vi "piano.vi"() -> ()   [LabVIEW 2016]
uses:
  <vilib>/userdefined/High Color/IMAQdx.ctl
  <vilib>/vision/driver/NI_Vision_Acquisition_Software.lvlib
  <vilib>/measure/NI_MABase.lvlib
panel:
  in  "Number of Erosion (Adv. Morphology 2)":i32=4
  in  "Threshold dedos":cluster{"Lower value":sgl, "Upper value":sgl}={"Lower value"=0.0, "Upper value"=20.0}
  in  "Threshold teclas":cluster{"Lower value":sgl, "Upper value":sgl}={"Lower value"=85.0, "Upper value"=255.0}
  in  "calibración":dbl
  out "Image":T1(plugin-control)
  out "Array":string[](array[string])
  in  "Stop (F)":bool
  out "Image Out":T1(plugin-control)
  # "100"
  # "Base y cámara fija:\n1- Configurar Mask\n2-configurar trheshold teclas blancas\n3-configurar threshold dedos\n4-configurar calibración (separación tolerable en pixeles\nde los centros de masa tecla y dedo)\n5-configurar número de teclas en código y orden de C a B"
  # "0"
  # "42"
  # "85"
  # "255"
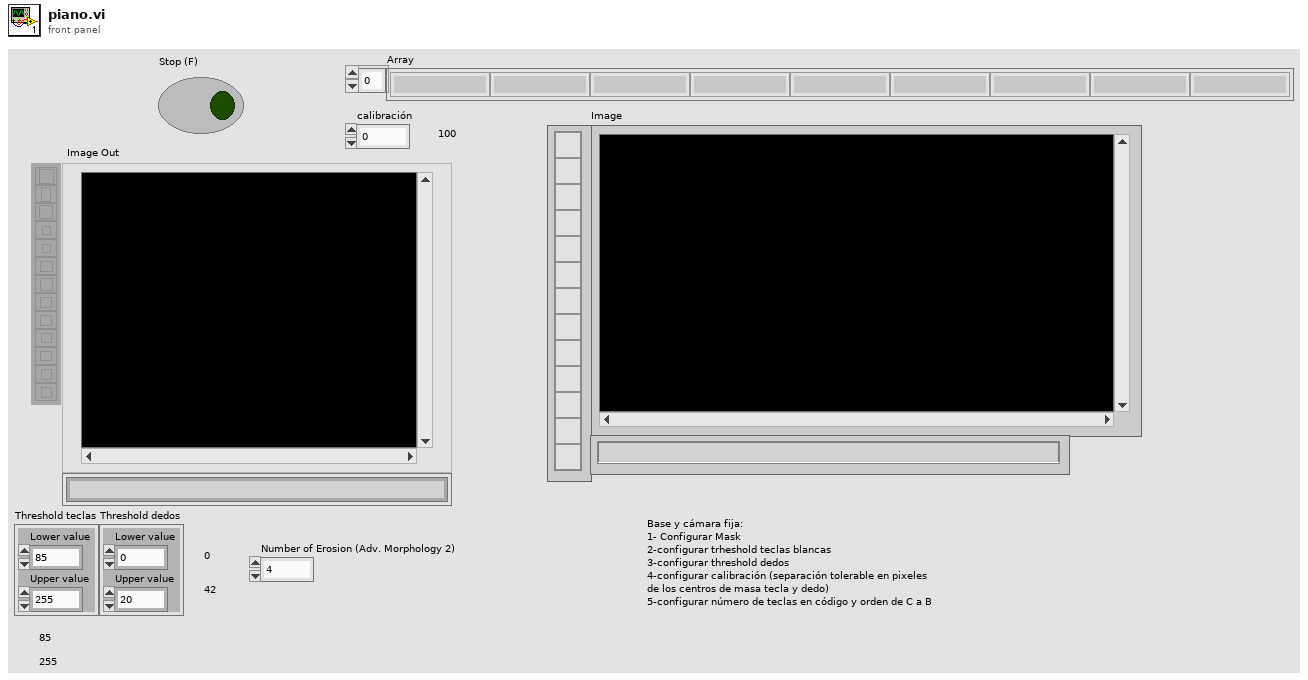
[diagram p1: front panel]
types:
  T1 = typedef "IMAQ Image.ctl" = refnum<image>
  T2 = typedef "Image Type" = u32
  T3 = typedef "IMAQdx.ctl" = refnum<k21>
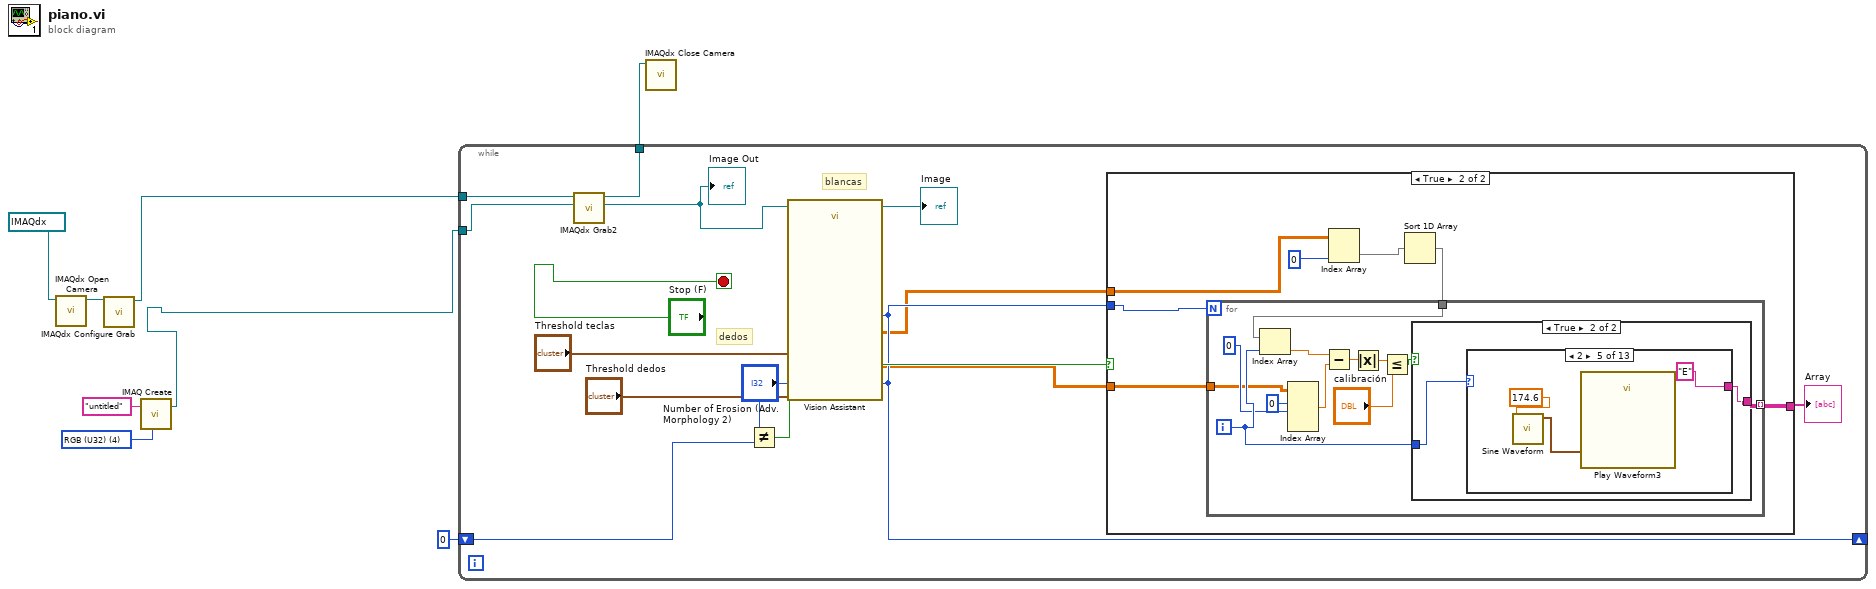
[diagram p0: block diagram]
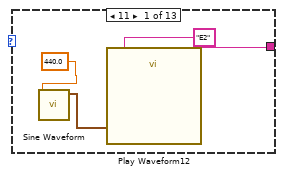
[diagram p4: hidden frame]
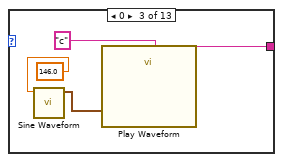
[diagram p6: hidden frame]
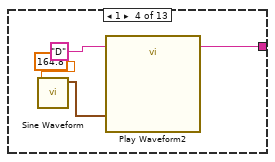
[diagram p7: hidden frame]
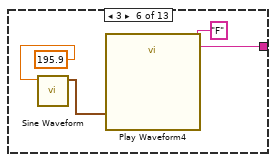
[diagram p8: hidden frame]
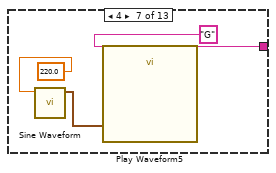
[diagram p9: hidden frame]
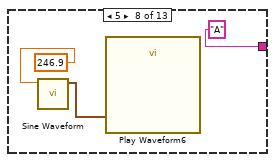
[diagram p10: hidden frame]
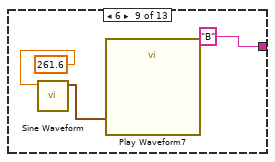
[diagram p11: hidden frame]
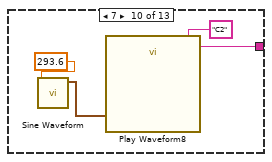
[diagram p12: hidden frame]
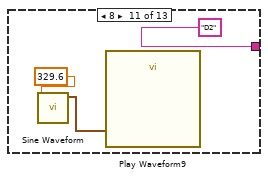
[diagram p13: hidden frame]
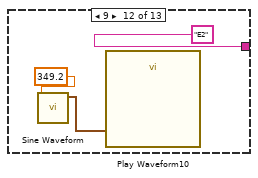
[diagram p14: hidden frame]
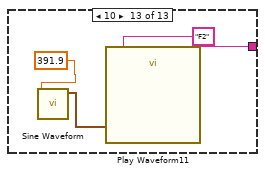
[diagram p15: hidden frame]
diagram:
  w1 = T2 4 items=["Grayscale (U8)", "Grayscale (I16)", "Grayscale (SGL)", "Complex (CSG)", "RGB (U32)", "HSL (U32)", "RGB (U64)", "Grayscale (U16)"] ("Image Type")
  n1 = call <vilib>:"IMAQdx Open Camera.vi"("Session In"=T3 "cam2") -> ("Session Out"=w8:T3)  [unwired: 9 in, 1 out]
  n2 = call <vilib>:"IMAQdx Configure Grab.vi"("Session In"=w8) -> ("Session Out"=w4:T3)  [unwired: 9 in, 1 out]
  n3 = call "IMAQ Create"("Image Name"="untitled", "Image Type"=w1) -> ("New Image"=w3:T1)  [unwired: 3 in, 1 out]
  n4 = while {
    tunnel: w4 -> [w19]
    tunnel: [w18] -> w7
    tunnel: w3 -> [w17]
    shift-right: [w15] -> _
    shift-left: 0 ("Number of Particles (Particle Analysis 1)") -> [w16]
    stop <- "Stop (F)" stop-if-true
    # "dedos"
    # "blancas"
    n5 = call <vilib>:"IMAQdx Grab2.vi"("Image In"=w17, "Session In"=w19) -> ("Image Out"=w13:T1, "Session Out"=w18:T3)  [unwired: 6 in, 2 out]
    "Image Out" <- w13
    n6 = call "Vision Assistant"("Image In"=w13, "Range (Threshold 1)"="Threshold teclas", "Range (Threshold 2)"="Threshold dedos", "Number of Erosion (Adv. Morphology 2)"="Number of Erosion (Adv. Morphology 2)") -> ("Image Out"=→"Image":T1, "Number of Particles (Particle Analysis 1)"=w15:i32, "Particle Measurements (Pixels) (Particle Analysis 1)"=w14:dbl[][], "Particle Measurements (Pixels) (Particle Analysis 2)"=w12:dbl[][])  [unwired: 18 in, 2 out]
    n7 = Not Equal?(x=w15, y=w16) -> (x != y?=w23:bool)
    n8 = case shown="True" w23 {
      tunnel: w14 -> [_ w27]
      tunnel: [_ w30] -> w22
      tunnel: w15 -> [_ w29]
      tunnel: w12 -> [_ w28]
      frame False {
      }
      frame True {
        n9 = Index Array(array=w27, index (col)=0 ("index (row)")) -> (element=w25:dbl[])  [unwired: 1 in]
        n10 = Sort 1D Array(array=w25) -> (sorted array=w24:dbl[])
        n11 = for {
          N: w29 -> [_]
          tunnel: [w42] -> w30 mode=indexing
          tunnel: w28 -> [w34]
          tunnel: w24 -> [w31]
          i -> [w41]
          n12 = Index Array(array=w31, index=w41) -> (element=w39:dbl)
          n13 = Index Array(array=w34, index (row) #1=0 ("disabled index (row)"), index (col) #1=0 ("index")) -> (element #1=w33:dbl)  [unwired: 2 in, 1 out]
          n14 = Subtract(x=w39, y=w33) -> (x-y=w38:dbl)
          n15 = Absolute Value(x=w38) -> (abs(x)=w36:dbl)
          n16 = Less Or Equal?(x=w36, y="calibración") -> (x <= y?=w37:bool)
          n17 = case shown="True" w37 {
            tunnel: w41 -> [_ w44]
            tunnel: [_ w43] -> w42
            frame False {
            }
            frame True {
              n18 = case shown="2" w44 {
                tunnel: ["E2" _ "c" "D" "E" "F" "G" "A" "B" "C2" "D2" "E2" "F2"] -> w43
                frame 11 {
                  n19 = call <vilib>:"Sine Waveform.vi"("frequency"=440.0) -> ("signal out"=w47:waveform(dbl))  [unwired: 9 in, 1 out]
                  n20 = call "Play Waveform12"("Data"=w47) -> ()  [unwired: 18 in, 1 out]
                }
                frame 12, Default {
                }
                frame 0 {
                  n21 = call <vilib>:"Sine Waveform.vi"("frequency"=146.0) -> ("signal out"=w48:waveform(dbl))  [unwired: 9 in, 1 out]
                  n22 = call "Play Waveform"("Data"=w48) -> ()  [unwired: 18 in, 1 out]
                }
                frame 1 {
                  n23 = call <vilib>:"Sine Waveform.vi"("frequency"=164.8) -> ("signal out"=w52:waveform(dbl))  [unwired: 9 in, 1 out]
                  n24 = call "Play Waveform2"("Data"=w52) -> ()  [unwired: 18 in, 1 out]
                }
                frame 2 {
                  n25 = call <vilib>:"Sine Waveform.vi"("frequency"=174.6) -> ("signal out"=w55:waveform(dbl))  [unwired: 9 in, 1 out]
                  n26 = call "Play Waveform3"("Data"=w55) -> ()  [unwired: 18 in, 1 out]
                }
                frame 3 {
                  n27 = call <vilib>:"Sine Waveform.vi"("frequency"=195.9) -> ("signal out"=w58:waveform(dbl))  [unwired: 9 in, 1 out]
                  n28 = call "Play Waveform4"("Data"=w58) -> ()  [unwired: 18 in, 1 out]
                }
                frame 4 {
                  n29 = call <vilib>:"Sine Waveform.vi"("frequency"=220.0) -> ("signal out"=w61:waveform(dbl))  [unwired: 9 in, 1 out]
                  n30 = call "Play Waveform5"("Data"=w61) -> ()  [unwired: 18 in, 1 out]
                }
                frame 5 {
                  n31 = call <vilib>:"Sine Waveform.vi"("frequency"=246.9) -> ("signal out"=w64:waveform(dbl))  [unwired: 9 in, 1 out]
                  n32 = call "Play Waveform6"("Data"=w64) -> ()  [unwired: 18 in, 1 out]
                }
                frame 6 {
                  n33 = call <vilib>:"Sine Waveform.vi"("frequency"=261.6) -> ("signal out"=w67:waveform(dbl))  [unwired: 9 in, 1 out]
                  n34 = call "Play Waveform7"("Data"=w67) -> ()  [unwired: 18 in, 1 out]
                }
                frame 7 {
                  n35 = call <vilib>:"Sine Waveform.vi"("frequency"=293.6) -> ("signal out"=w70:waveform(dbl))  [unwired: 9 in, 1 out]
                  n36 = call "Play Waveform8"("Data"=w70) -> ()  [unwired: 18 in, 1 out]
                }
                frame 8 {
                  n37 = call <vilib>:"Sine Waveform.vi"("frequency"=329.6) -> ("signal out"=w73:waveform(dbl))  [unwired: 9 in, 1 out]
                  n38 = call "Play Waveform9"("Data"=w73) -> ()  [unwired: 18 in, 1 out]
                }
                frame 9 {
                  n39 = call <vilib>:"Sine Waveform.vi"("frequency"=349.2) -> ("signal out"=w76:waveform(dbl))  [unwired: 9 in, 1 out]
                  n40 = call "Play Waveform10"("Data"=w76) -> ()  [unwired: 18 in, 1 out]
                }
                frame 10 {
                  n41 = call <vilib>:"Sine Waveform.vi"("frequency"=391.9) -> ("signal out"=w79:waveform(dbl))  [unwired: 9 in, 1 out]
                  n42 = call "Play Waveform11"("Data"=w79) -> ()  [unwired: 18 in, 1 out]
                }
              }
            }
          }
        }
      }
    }
    "Array" <- w22
  }
  n43 = call <vilib>:"IMAQdx Close Camera.vi"("Session In"=w7) -> ()  [unwired: 10 in, 1 out]
